vi "Vibration.vi"() -> ()   [LabVIEW 2012]
panel:
  out "?":enum32{"选项卡 1"}(tab)
  in  "AC/DC":bool
  in  "采样率(ksps)":T1(ring)=enum."105.468"
  in  "装置IP":string="192.168.1.16"
  in  "灵敏度4(mv/g)":i32=1 min=1
  in  "灵敏度3(mv/g)":i32=1 min=1
  in  "灵敏度2(mv/g)":i32=1 min=1
  in  "灵敏度1(mv/g)":i32=1 min=1
  in  "通道4":bool=TRUE
  in  "通道3":bool=TRUE
  in  "通道2":bool=TRUE
  in  "通道1":bool=TRUE
  out "?":dbl[][](graph)
  out "?":u16[](graph)
  in  "是否保存数据":bool
  in  "保存路径":path
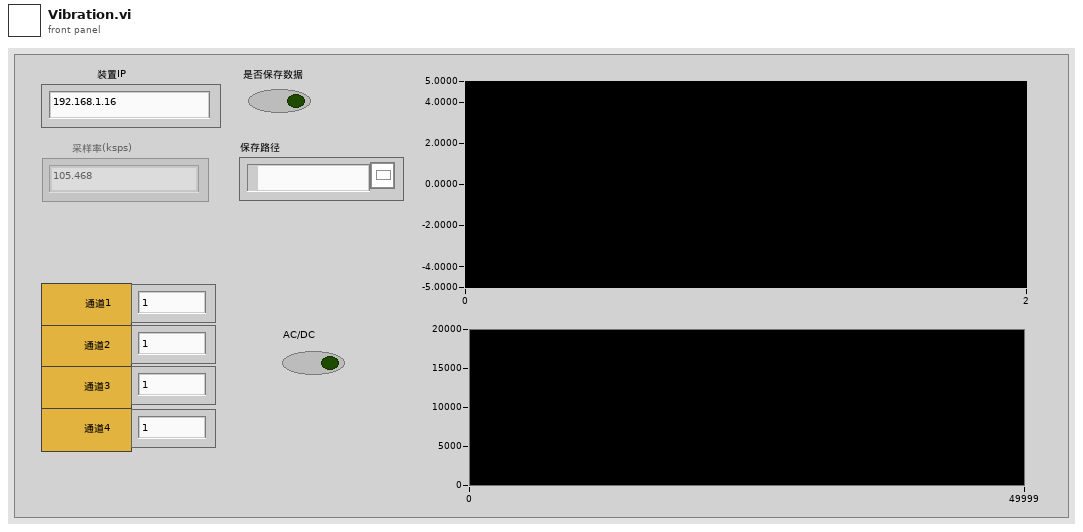
[diagram p1: front panel]
types:
  T1 = enum16{"", "105.468", "52.734", "35.156", "26.367", "21.094", "17.578", "15.067", "13.184", "11.719", "10.545"}
  T2 = cluster{"refnum":refnum<file>, "refnum":refnum<file>, "refnum":refnum<file>, "refnum":refnum<file>, "refnum":refnum<file>, "SavePath":path, "SAVE?":bool, "connection ID":refnum<k5>}
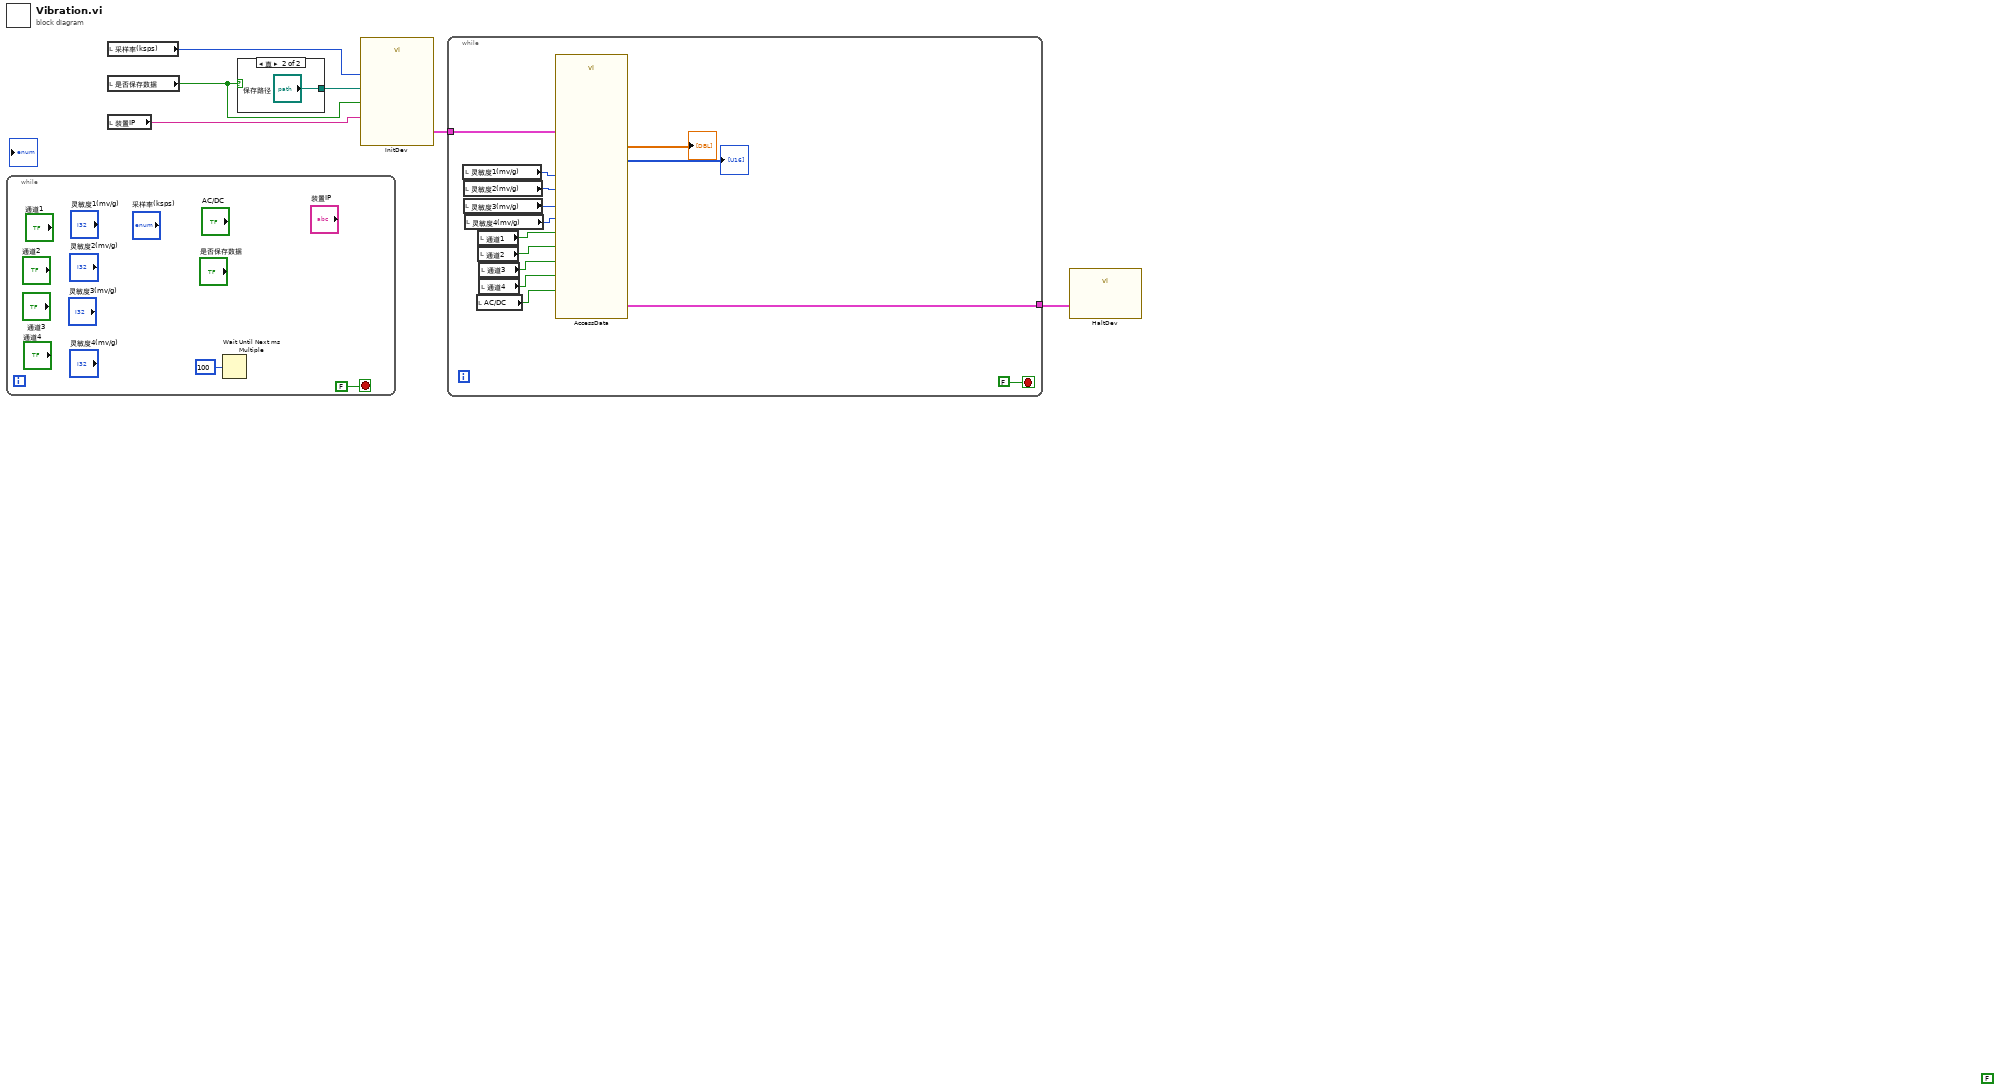
[diagram p0: block diagram]
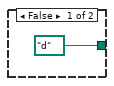
[diagram p2: hidden frame]
diagram:
  (unwired) FALSE
  n1 = while {
    stop <- FALSE stop-if-true
    n2 = Wait Until Next ms Multiple(millisecond multiple=u32 100 ("毫秒倍数")) -> ()  [unwired: 1 out]
  }
  n3 = local read "采样率(ksps)"() -> (w5:T1)
  n4 = local read "是否保存数据"() -> (w6:bool)
  n5 = local read "装置IP"() -> (w2:string)
  n6 = case shown="真" w6 {
    tunnel: [path "d:/" ("路径（使用对话框）") "保存路径"] -> w1
    frame False {
    }
    frame True {
    }
  }
  n7 = call "InitDev.vi"("SAVE?"=w6, "IP地址"=w2, "SampleRate"=w5, "SavePath"=w1) -> ("输出簇"=w3:T2)
  n8 = while {
    tunnel: w3 -> [w24]
    tunnel: [w23] -> w4
    stop <- FALSE stop-if-true
    n9 = local read "灵敏度1(mv/g)"() -> (w20:i32)
    n10 = local read "灵敏度2(mv/g)"() -> (w19:i32)
    n11 = local read "灵敏度3(mv/g)"() -> (w18:i32)
    n12 = local read "灵敏度4(mv/g)"() -> (w17:i32)
    n13 = local read "AC/DC"() -> (w12:bool)
    n14 = local read "通道1"() -> (w16:bool)
    n15 = local read "通道2"() -> (w15:bool)
    n16 = local read "通道3"() -> (w14:bool)
    n17 = local read "通道4"() -> (w13:bool)
    n18 = call "AccessData.vi"("Sensitivity1"=w20, "CH1Enable"=w16, "Sensitivity2"=w19, "CH2Enable"=w15, "Sensitivity3"=w18, "CH3Enable"=w14, "Sensitivity4"=w17, "CH4Enable"=w13, "输入簇"=w24, "RmOffset"=w12) -> ("VibrationWave"=→"?":dbl[][], "Speed"=→"?":u16[], "输出簇"=w23:T2)  [unwired: 2 in, 1 out]
  }
  n19 = call "HaltDev.vi"("输入簇"=w4) -> ()
